vi "Main.vi"() -> ()   [LabVIEW 2018]
doc: "This Continuous Measurement sample project is based on the Queued Message Handler template.\n\nThe Event Handling Loop generates messages based on user interface actions.\n\nThe Message Handling Loop processes messages generated by the Event Handling Loop, or by other messages. There are also Acquisition and Logging message handling loop subVIs, and a chart updating loop."
uses:
  Settings/Settings.ctl
  Acquisition/Hardware Configuration.ctl
  Logging/Logging Configuration.ctl
  controls/UI Data.ctl
  controls/UI State.ctl
  support/Message Queue/Enqueue Message (Single).vi
  <vilib>/Utility/error.llb/Error Cluster From Error Code.vi
  <vilib>/ErrorRing/Error Ring.xnode
  Acquisition/Acquisition.lvlib
  Logging/Logging.lvlib
  Settings/Settings.lvlib
  support/User Event - Stop/User Event - Stop.lvlib
  support/Message Queue/Message Queue.lvlib
panel:
  out "Data":waveform(dbl)[](graph)
  in  "Force Trigger":bool
  in  "Settings":bool
  in  "Start":bool
  in  "Stop":bool
  out "Status":string
  in  "Exit":bool
  # "Continuous Measurement and Logging (NI-DAQmx)"
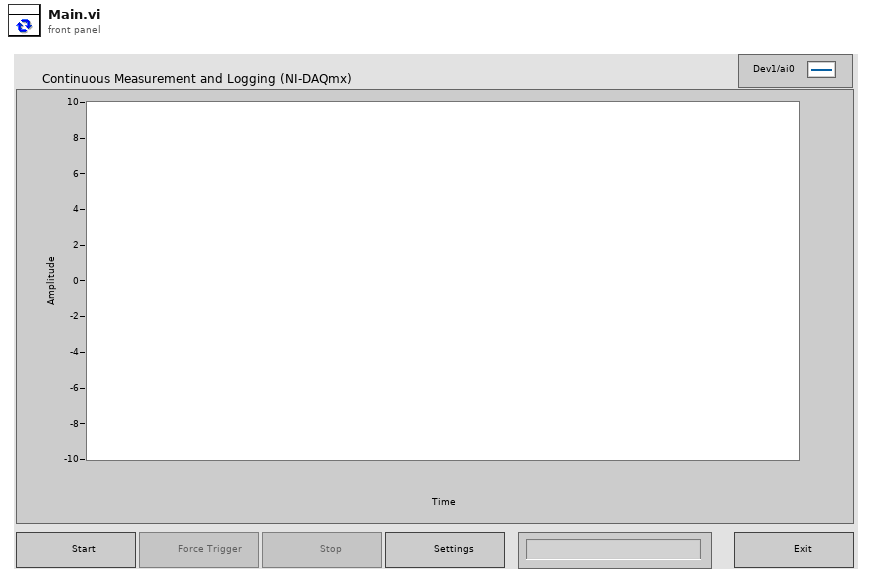
[diagram p1: front panel]
types:
  T1 = typedef "UI State.ctl" = enum16{"Idle", "Acquiring and Logging", "Waiting for Exit", "Waiting for Exit (Acq Stopped)", "Waiting for Exit (Log Stopped)", "Waiting for Stop", "Waiting for Stop (Acq Stopped)", "Waiting for Stop (Log Stopped)"}
  T2 = typedef "UI Data.ctl" = cluster{"Start Ref":refnum<vi>, "Trigger Ref":refnum<vi>, "Stop Ref":refnum<vi>, "Settings Ref":refnum<vi>, "Status Ref":refnum<vi>, "Exit Ref":refnum<vi>, "Data Ref":refnum<vi>}
  T3 = typedef "Settings.lvlib/Settings.ctl" = cluster{"Hardware Configuration":T4, "Logging Configuration":T5}
  T4 = typedef "Acquisition.lvlib/Hardware Configuration.ctl" = cluster{"DAQmx Channel":tag, "Max Input":dbl, "Min Input":dbl, "Sample Rate":dbl, "DAQmx Task":refnum<k21>}
  T5 = typedef "Logging.lvlib/Logging Configuration.ctl" = cluster{"Log File Base Path":path, "TDMS File Reference":refnum<k34>, "Samples to Save":u32, "Trigger - Time":u32, "Trigger - Threshold":dbl, "Trigger - Channel":u32, "Enable Time Trigger":bool, "Enable Threshold Trigger":bool, "Always Log":bool}
  T6 = typedef "Message Queue.lvlib/All Message Queues.ctl" = cluster{"UI":refnum<queue>, "Acquisition":refnum<queue>, "Logging":refnum<queue>}
  T7 = enum8{"Enabled", "Disabled", "Disabled and Grayed Out"}
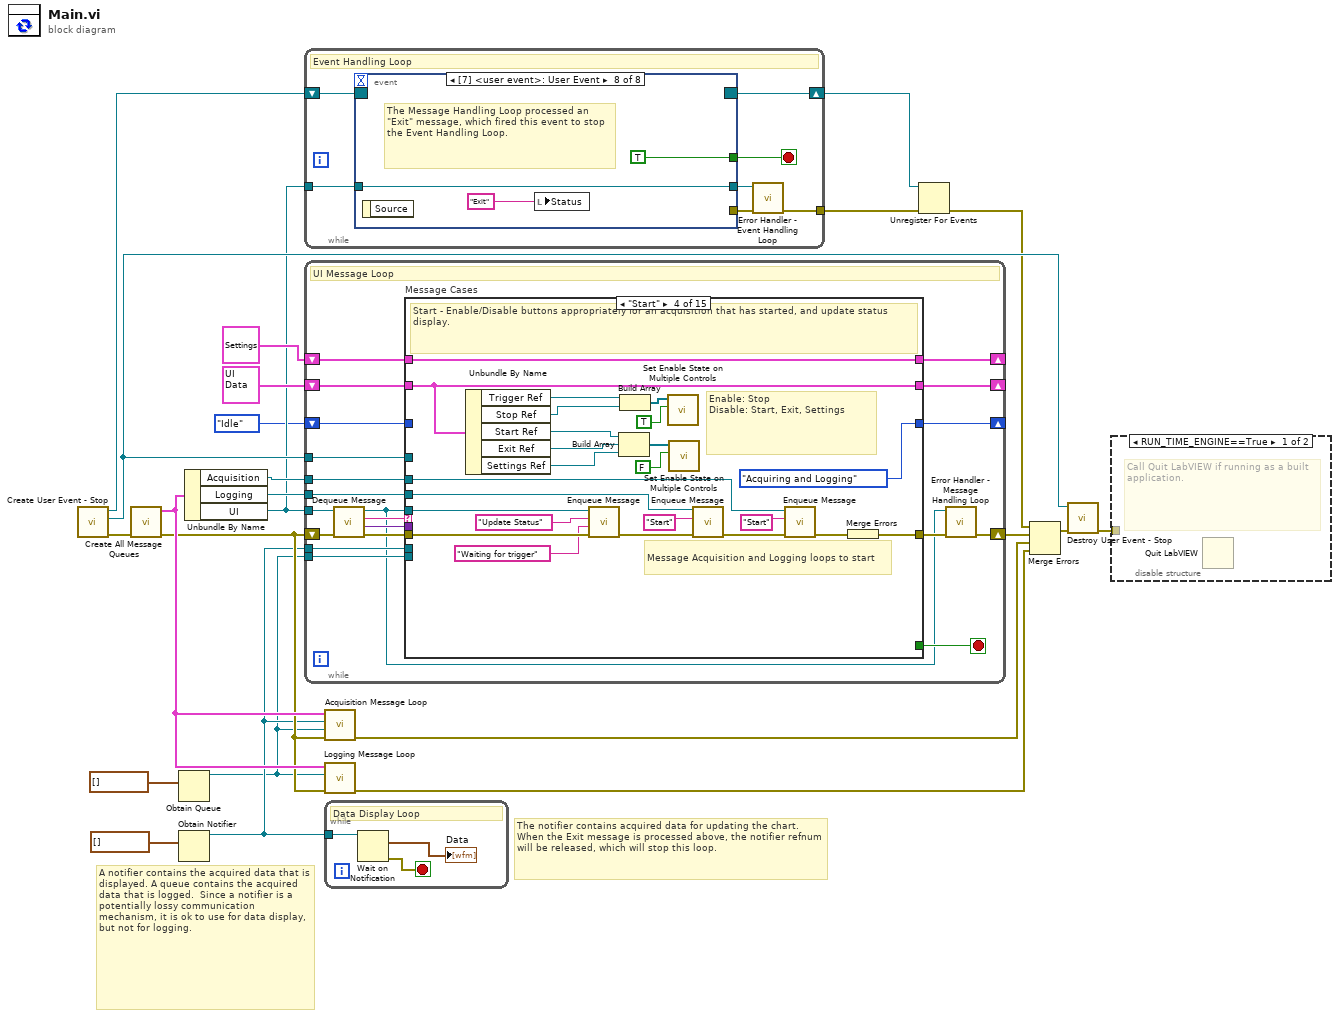
[diagram p0: block diagram]
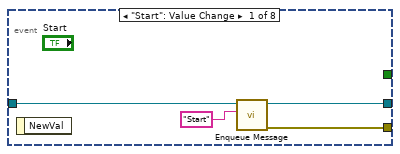
[diagram p3: hidden frame]
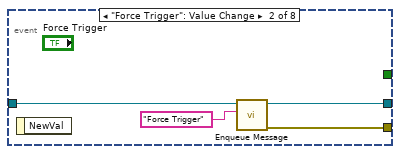
[diagram p4: hidden frame]
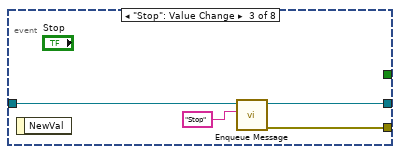
[diagram p5: hidden frame]
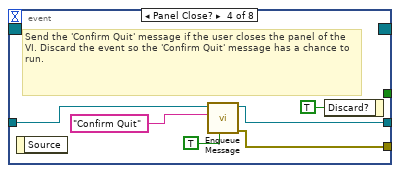
[diagram p6: hidden frame]
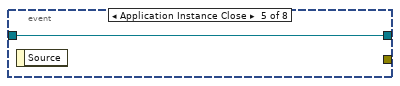
[diagram p7: hidden frame]
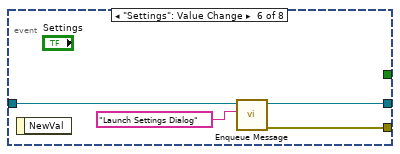
[diagram p8: hidden frame]
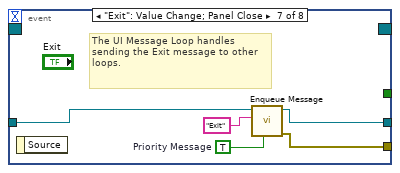
[diagram p9: hidden frame]
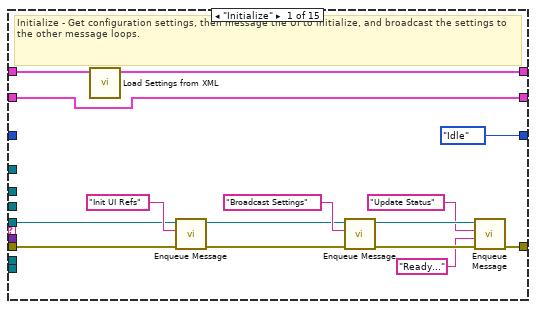
[diagram p10: hidden frame]
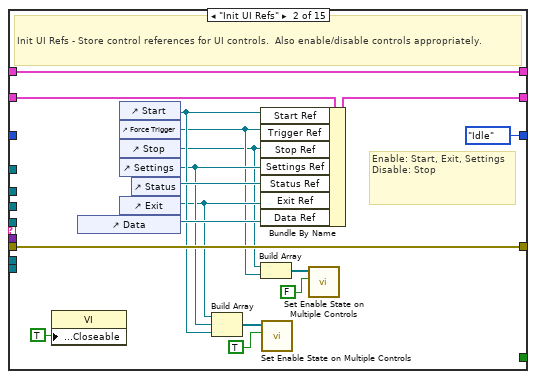
[diagram p11: hidden frame]
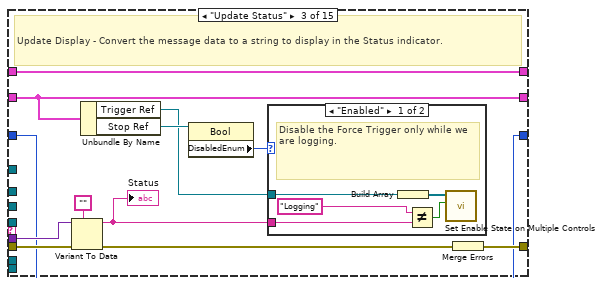
[diagram p12: hidden frame]
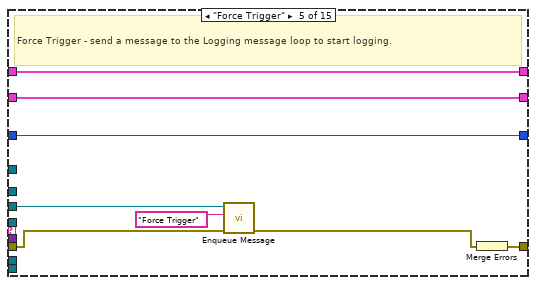
[diagram p14: hidden frame]
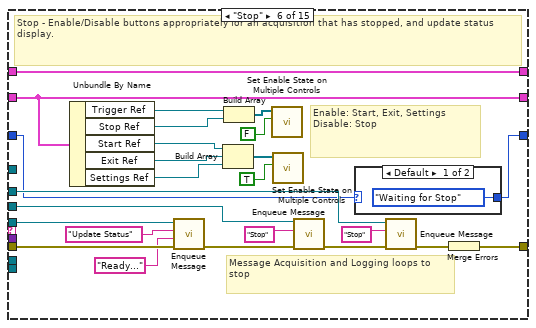
[diagram p15: hidden frame]
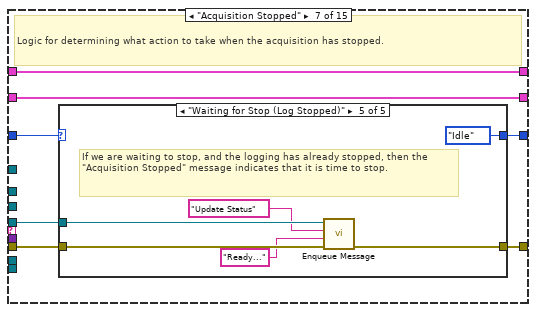
[diagram p17: hidden frame]
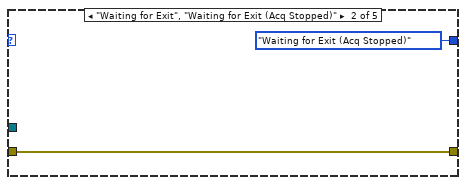
[diagram p19: hidden frame]
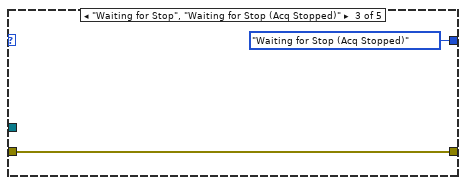
[diagram p20: hidden frame]
diagram:
  # "A notifier contains the acquired data that is displayed. A queue contains the acquired data that is logged.  Since a notifier is a potentially lossy communication mechanism, it is ok to use for data display, but not for logging."
  # "The notifier contains acquired data for updating the chart. When the Exit message is processed above, the notifier refnum will be released, which will stop this loop."
  n1 = call "Create User Event - Stop.vi"() -> ("error out"=w17:errorcluster, "User Event - Stop"=w19:refnum<user-event>, "Stop Event Registration Refnum"=w20:refnum<event-registration>)  [unwired: 9 in]
  n2 = call "Create All Message Queues.vi"("error in (no error)"=w17) -> ("error out"=w14:errorcluster, "Message Queues out"=w16:T6)  [unwired: 9 in]
  n3 = Obtain Queue(element data type=waveform(dbl)[] []) -> (queue out=w3:refnum<queue>)  [unwired: 4 in, 2 out]
  n4 = Obtain Notifier(notification data type=waveform(dbl)[] []) -> (notifier out=w5:refnum<notifier>)  [unwired: 3 in, 2 out]
  n5 = Unbundle By Name(w16) -> ("Acquisition"=w9:refnum<queue>, "Logging"=w8:refnum<queue>, "UI"=w7:refnum<queue>)
  n6 = while {
    tunnel: w7 -> [w29]
    tunnel: [w24] -> w22
    shift-right: [w28] -> w11
    shift-left: w20 -> [w30]
    stop <- w27 stop-if-true
    # "Event Handling Loop"
    n7 = event shown="[7] <user event>: User Event" {
      selector: w30 -> [_ _ _ _ _ _ _ _]
      dyn-events: [_ _ _ _ _ _ _ _] -> w28
      timeout: _ -> [_ _ _ _ _ _ _ _]
      tunnel: [_ _ _ _ _ _ _ TRUE ("Discard?")] -> w27
      tunnel: w29 -> [w32 w37 w41 w48 w49 w51 w55 w59]
      tunnel: [w34 w36 w40 w43 _ w53 w58 _] -> w25
      tunnel: [w31 w35 w39 w44 w49 w50 w54 w59] -> w26
      event "Start": Value Change {
        n8 = event-data() -> ()  [unwired: 1 in, 1 out]
        n9 = call-poly "Enqueue Message.vi"("Message"="Start", "Message Queue"=w32) -> ("error out"=w34:errorcluster, "dup Message Queue"=w31:refnum<queue>)  [unwired: 8 in]
      }
      event "Force Trigger": Value Change {
        n10 = event-data() -> ()  [unwired: 1 in, 1 out]
        n11 = call-poly "Enqueue Message.vi"("Message"="Force Trigger", "Message Queue"=w37) -> ("error out"=w36:errorcluster, "dup Message Queue"=w35:refnum<queue>)  [unwired: 8 in]
      }
      event "Stop": Value Change {
        n12 = event-data() -> ()  [unwired: 1 in, 1 out]
        n13 = call-poly "Enqueue Message.vi"("Message"="Stop", "Message Queue"=w41) -> ("error out"=w40:errorcluster, "dup Message Queue"=w39:refnum<queue>)  [unwired: 8 in]
      }
      event Panel Close? {
        # "Send the 'Confirm Quit' message if the user closes the panel of the VI. Discard the event so the 'Confirm Quit' message has a chance to run."
        n14 = event-data() -> ()  [unwired: 1 in, 1 out]
        n15 = call-poly "Enqueue Message.vi"("Priority Message? (F)"=TRUE, "Message"="Confirm Quit", "Message Queue"=w48) -> ("error out"=w43:errorcluster, "dup Message Queue"=w44:refnum<queue>)  [unwired: 7 in]
        n16 = event-data("Discard?"=TRUE) -> ()  [unwired: 1 in, 1 out]
      }
      event Application Instance Close {
        n17 = event-data() -> ()  [unwired: 1 in, 1 out]
      }
      event "Settings": Value Change {
        n18 = event-data() -> ()  [unwired: 1 in, 1 out]
        n19 = call-poly "Enqueue Message.vi"("Message"="Launch Settings Dialog", "Message Queue"=w51) -> ("error out"=w53:errorcluster, "dup Message Queue"=w50:refnum<queue>)  [unwired: 8 in]
      }
      event "Exit": Value Change; Panel Close {
        w56 = TRUE  # Priority Message
        # "The UI Message Loop handles sending the Exit message to other loops."
        n20 = event-data() -> ()  [unwired: 1 in, 1 out]
        n21 = call-poly "Enqueue Message.vi"("Priority Message? (F)"=w56, "Message"="Exit", "Message Queue"=w55) -> ("error out"=w58:errorcluster, "dup Message Queue"=w54:refnum<queue>)  [unwired: 7 in]
      }
      event User Event {
        # "The Message Handling Loop processed an \"Exit\" message, which fired this event to stop the Event Handling Loop."
        n22 = event-data() -> ()  [unwired: 1 in, 1 out]
        n23 = local write "Status"("Exit" ("Exit String")) -> ()
      }
    }
    n24 = call "Error Handler - Event Handling Loop.vi"("error in (no error)"=w25, "Message Queue"=w26) -> ("dup error in"=w24:errorcluster)  [unwired: 8 in, 1 out]
  }
  n25 = while {
    tunnel: w7 -> [w75]
    tunnel: w19 -> [w80]
    shift-right: [w65] -> w23
    shift-left: w14 -> [w79]
    shift-right: [w74] -> _
    shift-left: T3 {"Hardware Configuration"={"DAQmx Channel"="", "Max Input"=0.0, "Min Input"=0.0, "Sample Rate"=0.0, "DAQmx Task"=""}, "Logging Configuration"={"Log File Base Path"=path "", "TDMS File Reference"=refnum, "Samples to Save"=0, "Trigger - Time"=0, "Trigger - Threshold"=0.0, "Trigger - Channel"=0, "Enable Time Trigger"=FALSE, "Enable Threshold Trigger"=FALSE, "Always Log"=FALSE}} ("Settings") -> [w73]
    shift-right: [w71] -> _
    shift-left: T2 {"Start Ref"=refnum, "Trigger Ref"=refnum, "Stop Ref"=refnum, "Settings Ref"=refnum, "Status Ref"=refnum, "Exit Ref"=refnum, "Data Ref"=refnum} ("Measurement UI Controls") -> [w72]
    tunnel: w9 -> [w70]
    tunnel: w8 -> [w69]
    tunnel: w5 -> [w68]
    tunnel: w3 -> [w67]
    shift-right: [w62] -> _
    shift-left: UI_State."Idle" ("UI State") -> [w63]
    stop <- w81 stop-if-true
    # "UI Message Loop"
    n26 = call "Dequeue Message.vi"("error in (no error)"=w79, "Message Queue"=w75) -> ("error out"=w78:errorcluster, "Message Data"=w76:variant, "Message"=w77:string, "dup Message Queue"=w64:refnum<queue>)  [unwired: 6 in]
    n27 = case "Message Cases" shown="\"Start\"" w77 {
      selector: w77 -> [_ _ _ _ _ _ _ _ _ _ _ _ _ _ w332]
      tunnel: w64 -> [w86 _ _ w153 _ w186 w190 w215 _ w257 w272 w282 w315 _ _]
      tunnel: w78 -> [w85 w113 w124 w152 w159 w185 w192 w217 w245 w259 w276 w281 w323 w330 _]
      tunnel: [w92 w113 w125 w154 w162 w187 w191 w216 w251 w254 w267 w280 w324 w329 w333] -> w66
      tunnel: [_ _ _ _ _ _ _ _ _ _ _ _ TRUE _ _] -> w81
      tunnel: w76 -> [_ _ w123 _ _ _ _ _ _ _ w275 _ _ _ _]
      tunnel: w80 -> [_ _ _ _ _ _ _ _ _ _ _ _ w322 _ _]
      tunnel: [w95 w112 w120 w151 w161 w184 w196 w221 w249 w256 w278 w285 w320 w328 w335] -> w74
      tunnel: w73 -> [w96 w112 w120 w151 w161 w184 w196 w221 w249 w260 w278 w285 w320 w328 w335]
      tunnel: w72 -> [w88 w111 w119 w148 w160 w181 w195 w220 w243 w253 w277 w284 w318 w327 w334]
      tunnel: [w88 w110 w119 w148 w160 w181 w195 w220 w243 w253 w277 w284 w318 w327 w334] -> w71
      tunnel: w70 -> [_ _ _ w135 _ w168 _ _ w242 _ _ _ w317 _ _]
      tunnel: w69 -> [_ _ _ w138 w156 w171 _ _ w241 _ _ _ w316 _ _]
      tunnel: w68 -> [_ _ _ _ _ _ _ _ _ _ _ _ w314 _ _]
      tunnel: w67 -> [_ _ _ _ _ _ _ _ _ _ _ _ w310 _ _]
      tunnel: w63 -> [_ _ w114 _ w155 w164 w194 w219 w240 w252 w266 w283 _ w326 w331]
      tunnel: [UI_State."Idle" ("UI State") UI_State."Idle" ("UI State") w114 UI_State."Acquiring and Logging" ("UI State") w155 w163 w193 w218 w240 w252 w266 w279 UI_State."Idle" ("UI State") w326 w331] -> w62
      frame "Initialize" {
        # "Initialize - Get configuration settings, then message the UI to initialize, and broadcast the settings to the other message loops."
        n28 = call "Load Settings from XML.vi"("Settings in"=w96) -> ("Settings out"=w95:T3)  [unwired: 9 in, 1 out]
        n29 = call-poly "Enqueue Message.vi"("error in (no error)"=w85, "Message"="Init UI Refs", "Message Queue"=w86) -> ("error out"=w83:errorcluster, "dup Message Queue"=w84:refnum<queue>)  [unwired: 7 in]
        n30 = call-poly "Enqueue Message.vi"("error in (no error)"=w83, "Message"="Broadcast Settings", "Message Queue"=w84) -> ("error out"=w94:errorcluster, "dup Message Queue"=w93:refnum<queue>)  [unwired: 7 in]
        n31 = call-poly "Enqueue Message.vi"("error in (no error)"=w94, "Message Data"="Ready..." ("Ready..."), "Message"="Update Status", "Message Queue"=w93) -> ("error out"=w92:errorcluster)  [unwired: 6 in, 1 out]
      }
      frame "Init UI Refs" {
        # "Enable: Start, Exit, Settings\nDisable: Stop"
        # "Init UI Refs - Store control references for UI controls.  Also enable/disable controls appropriately."
        n32 = property class="VI"("Front Panel.Closeable"=TRUE ("Front Panel Window:Closeable")) -> ()  [unwired: 2 in, 2 out]
        n33 = control-ref of="Data"() -> (w106:refnum<vi>)
        n34 = control-ref of="Start"() -> (w105:refnum<vi>)
        n35 = control-ref of="Force Trigger"() -> (w100:refnum<vi>)
        n36 = control-ref of="Stop"() -> (w99:refnum<vi>)
        n37 = control-ref of="Settings"() -> (w102:refnum<vi>)
        n38 = control-ref of="Exit"() -> (w101:refnum<vi>)
        n39 = control-ref of="Status"() -> (w107:refnum<vi>)
        n40 = Build Array(w101, w102, w105) -> (w104:refnum<vi>[])
        n41 = Bundle By Name(cluster=w111, "Start Ref"=w105, "Trigger Ref"=w100, "Stop Ref"=w99, "Settings Ref"=w102, "Status Ref"=w107, "Exit Ref"=w101, "Data Ref"=w106) -> (w110:T2)
        n42 = Build Array(w99, w100) -> (w98:refnum<vi>[])
        n43 = call "Set Enable State on Multiple Controls.vi"("Enable?"=TRUE, "Controls"=w104) -> ()  [unwired: 10 in]
        n44 = call "Set Enable State on Multiple Controls.vi"("Enable?"=FALSE, "Controls"=w98) -> ()  [unwired: 10 in]
      }
      frame "Update Status" {
        # "Update Display - Convert the message data to a string to display in the Status indicator."
        n45 = Variant To Data(error in=w124, type="", Variant=w123) -> (data=w116:string, error out=w121:errorcluster)
        "Status" <- w116
        n46 = Unbundle By Name(w119) -> ("Trigger Ref"=w115:refnum<vi>, "Stop Ref"=w118:refnum<vi>)
        n47 = property class="Bool"(reference=w118) -> ("DisabledEnum"=w117:T7)  [unwired: 1 in, 2 out]
        n48 = case shown="\"Enabled\"" w117 {
          tunnel: w116 -> [w128 _]
          tunnel: w115 -> [w129 _]
          frame "Enabled" {
            # "Disable the Force Trigger only while we are logging."
            n49 = Build Array(w129) -> (w130:refnum<vi>[])
            n50 = Not Equal?(x="Logging" ("Logging"), y=w128) -> (x != y?=w126:bool)
            n51 = call "Set Enable State on Multiple Controls.vi"("Enable?"=w126, "Controls"=w130) -> ()  [unwired: 10 in]
          }
          frame "Disabled", Default {
          }
        }
        n52 = Merge Errors(w121) -> (w125:errorcluster)
      }
      frame "Start" {
        # "Message Acquisition and Logging loops to start"
        # "Enable: Stop\nDisable: Start, Exit, Settings"
        # "Start - Enable/Disable buttons appropriately for an acquisition that has started, and update status display."
        n53 = Unbundle By Name(w148) -> ("Trigger Ref"=w132:refnum<vi>, "Stop Ref"=w133:refnum<vi>, "Start Ref"=w143:refnum<vi>, "Exit Ref"=w142:refnum<vi>, "Settings Ref"=w141:refnum<vi>)
        n54 = call-poly "Enqueue Message.vi"("error in (no error)"=w152, "Message Data"="Waiting for trigger" ("Waiting for trigger"), "Message"="Update Status", "Message Queue"=w153) -> ("error out"=w140:errorcluster)  [unwired: 6 in, 1 out]
        n55 = Build Array(w143, w142, w141) -> (w146:refnum<vi>[])
        n56 = Build Array(w132, w133) -> (w145:refnum<vi>[])
        n57 = call "Set Enable State on Multiple Controls.vi"("Enable?"=TRUE, "Controls"=w145) -> ()  [unwired: 10 in]
        n58 = call "Set Enable State on Multiple Controls.vi"("Enable?"=FALSE, "Controls"=w146) -> ()  [unwired: 10 in]
        n59 = call-poly "Enqueue Message.vi"("error in (no error)"=w140, "Message"="Start", "Message Queue"=w138) -> ("error out"=w137:errorcluster)  [unwired: 7 in, 1 out]
        n60 = call-poly "Enqueue Message.vi"("error in (no error)"=w137, "Message"="Start", "Message Queue"=w135) -> ("error out"=w136:errorcluster)  [unwired: 7 in, 1 out]
        n61 = Merge Errors(w136) -> (w154:errorcluster)
      }
      frame "Force Trigger" {
        # "Force Trigger - send a message to the Logging message loop to start logging."
        n62 = call-poly "Enqueue Message.vi"("error in (no error)"=w159, "Message"="Force Trigger", "Message Queue"=w156) -> ("error out"=w158:errorcluster)  [unwired: 7 in, 1 out]
        n63 = Merge Errors(w158) -> (w162:errorcluster)
      }
      frame "Stop" {
        # "Message Acquisition and Logging loops to stop"
        # "Enable: Start, Exit, Settings\nDisable: Stop"
        # "Stop - Enable/Disable buttons appropriately for an acquisition that has stopped, and update status display."
        n64 = Unbundle By Name(w181) -> ("Trigger Ref"=w165:refnum<vi>, "Stop Ref"=w166:refnum<vi>, "Start Ref"=w176:refnum<vi>, "Exit Ref"=w175:refnum<vi>, "Settings Ref"=w174:refnum<vi>)
        n65 = call-poly "Enqueue Message.vi"("error in (no error)"=w185, "Message Data"="Ready..." ("Ready..."), "Message"="Update Status", "Message Queue"=w186) -> ("error out"=w173:errorcluster)  [unwired: 6 in, 1 out]
        n66 = Build Array(w176, w175, w174) -> (w179:refnum<vi>[])
        n67 = Build Array(w165, w166) -> (w178:refnum<vi>[])
        n68 = call "Set Enable State on Multiple Controls.vi"("Enable?"=FALSE, "Controls"=w178) -> ()  [unwired: 10 in]
        n69 = call "Set Enable State on Multiple Controls.vi"("Enable?"=TRUE, "Controls"=w179) -> ()  [unwired: 10 in]
        n70 = call-poly "Enqueue Message.vi"("error in (no error)"=w173, "Message"="Stop", "Message Queue"=w171) -> ("error out"=w170:errorcluster)  [unwired: 7 in, 1 out]
        n71 = case shown="Default" w164 {
          selector: w164 -> [_ w189]
          tunnel: [UI_State."Waiting for Stop" ("UI State") w189] -> w163
          frame Default {
          }
          frame "Waiting for Exit" {
          }
        }
        n72 = call-poly "Enqueue Message.vi"("error in (no error)"=w170, "Message"="Stop", "Message Queue"=w168) -> ("error out"=w169:errorcluster)  [unwired: 7 in, 1 out]
        n73 = Merge Errors(w169) -> (w187:errorcluster)
      }
      frame "Acquisition Stopped" {
        # "Logic for determining what action to take when the acquisition has stopped."
        n74 = case shown="\"Waiting for Stop (Log Stopped)\"" w194 {
          selector: w194 -> [w198 _ _ _ _]
          tunnel: [w198 UI_State."Waiting for Exit (Acq Stopped)" ("UI State") UI_State."Waiting for Stop (Acq Stopped)" ("UI State") UI_State."Idle" ("UI State") UI_State."Idle" ("UI State")] -> w193
          tunnel: w192 -> [w197 w199 w201 w207 w213]
          tunnel: [w197 w199 w201 w206 w212] -> w191
          tunnel: w190 -> [_ _ _ w205 w211]
          frame Default {
          }
          frame "Waiting for Exit", "Waiting for Exit (Acq Stopped)" {
          }
          frame "Waiting for Stop", "Waiting for Stop (Acq Stopped)" {
          }
          frame "Waiting for Exit (Log Stopped)" {
            # "If we are waiting to exit, and the logging has already stopped, then the \"Acquisition Stopped\" message indicates that it is time to exit."
            n75 = call-poly "Enqueue Message.vi"("Priority Message? (F)"=TRUE, "error in (no error)"=w207, "Message"="Exit", "Message Queue"=w205) -> ("error out"=w206:errorcluster)  [unwired: 6 in, 1 out]
          }
          frame "Waiting for Stop (Log Stopped)" {
            # "If we are waiting to stop, and the logging has already stopped, then the \"Acquisition Stopped\" message indicates that it is time to stop."
            n76 = call-poly "Enqueue Message.vi"("error in (no error)"=w213, "Message Data"="Ready..." ("Message"), "Message"="Update Status", "Message Queue"=w211) -> ("error out"=w212:errorcluster)  [unwired: 6 in, 1 out]
          }
        }
      }
      frame "Logging Stopped" {
        # "Logic for determining what action to take when the logging has stopped."
        n77 = case shown="\"Waiting for Stop (Acq Stopped)\"" w219 {
          selector: w219 -> [w223 _ _ _ _]
          tunnel: [w223 UI_State."Waiting for Exit (Log Stopped)" ("UI State") UI_State."Waiting for Stop (Log Stopped)" ("UI State") UI_State."Idle" ("UI State") UI_State."Idle" ("UI State")] -> w218
          tunnel: w217 -> [w222 w224 w226 w232 w238]
          tunnel: [w222 w224 w226 w231 w237] -> w216
          tunnel: w215 -> [_ _ _ w230 w236]
          frame Default {
          }
          frame "Waiting for Exit", "Waiting for Exit (Log Stopped)" {
          }
          frame "Waiting for Stop", "Waiting for Stop (Log Stopped)" {
          }
          frame "Waiting for Exit (Acq Stopped)" {
            # "If we are waiting to exit, and the acquisition has already stopped, then the \"Logging Stopped\" message indicates that it is time to exit."
            n78 = call-poly "Enqueue Message.vi"("Priority Message? (F)"=TRUE, "error in (no error)"=w232, "Message"="Exit", "Message Queue"=w230) -> ("error out"=w231:errorcluster)  [unwired: 6 in, 1 out]
          }
          frame "Waiting for Stop (Acq Stopped)" {
            # "If we are waiting to stop, and the acquisition has already stopped, then the \"Logging Stopped\" message indicates that it is time to stop."
            n79 = call-poly "Enqueue Message.vi"("error in (no error)"=w238, "Message Data"="Ready..." ("Message"), "Message"="Update Status", "Message Queue"=w236) -> ("error out"=w237:errorcluster)  [unwired: 6 in, 1 out]
          }
        }
      }
      frame "Broadcast settings" {
        w244 = "Update Settings" ("Message")
        # "Send the 'Update Settings' message to the Logging and Acquisition message loops."
        n80 = Unbundle By Name(w249) -> ("Hardware Configuration"=w248:T4, "Logging Configuration"=w247:T5)
        n81 = call-poly "Enqueue Message.vi"("Message Data"=w248, "Message"=w244, "Message Queue"=w242) -> ("error out"=w250:errorcluster)  [unwired: 7 in, 1 out]
        n82 = call-poly "Enqueue Message.vi"("error in (no error)"=w250, "Message Data"=w247, "Message"=w244, "Message Queue"=w241) -> ("error out"=w246:errorcluster)  [unwired: 6 in, 1 out]
        n83 = Merge Errors(w246, w245) -> (w251:errorcluster)
      }
      frame "Launch Settings Dialog" {
        # "Launch the Settings Dialog when the user clicks the 'Settings' button."
        n84 = call "Settings Dialog.vi"("error in (no error)"=w259, "Settings in"=w260) -> ("error out"=w255:errorcluster, "Cancelled?"=w258:bool, "Settings out"=w256:T3)  [unwired: 6 in, 1 out]
        n85 = case shown="False" w258 {
          tunnel: w257 -> [w264 _]
          tunnel: w255 -> [w263 w265]
          tunnel: [w262 w265] -> w254
          frame False {
            n86 = call-poly "Enqueue Message.vi"("error in (no error)"=w263, "Message"="Broadcast Settings", "Message Queue"=w264) -> ("error out"=w262:errorcluster)  [unwired: 7 in, 1 out]
          }
          frame True {
          }
        }
      }
      frame "Error" {
        # "Error - Check the error message data and respond accordingly. This message is sent by the \"Error Handler\" VIs at the end of each loop in this application."
        n87 = Variant To Data(error in=w276, type=errorcluster {"status"=FALSE, "code"=0, "source"=""} ("error out"), Variant=w275) -> (data=w273:errorcluster, error out=w269:errorcluster)
        n88 = call <vilib>:"Simple Error Handler.vi"("error in (no error)"=w273) -> ()  [unwired: 4 in, 5 out]
        n89 = call-poly "Enqueue Message.vi"("Priority Message? (F)"=TRUE, "Message"="Exit", "Message Queue"=w272) -> ("error out"=w268:errorcluster)  [unwired: 7 in, 1 out]
        n90 = Merge Errors(w268, w269) -> (w267:errorcluster)
      }
      frame "Confirm Quit" {
        # "Confirm Quit - Message that can confirm whether or not the user wants to exit the application."
        n91 = case shown="\"Acquiring and Logging\"" w283 {
          tunnel: w282 -> [w290 w296]
          tunnel: w281 -> [w289 w294]
          tunnel: [w286 w293] -> w280
          tunnel: [UI_State."Idle" ("UI State") w292] -> w279
          frame Default {
            # "If 'Confirm Quit' comes in while the system is idle, there is no need for a confirmation message."
            n92 = call-poly "Enqueue Message.vi"("Priority Message? (F)"=TRUE, "error in (no error)"=w289, "Message"="Exit", "Message Queue"=w290) -> ("error out"=w286:errorcluster)  [unwired: 6 in, 1 out]
          }
          frame "Acquiring and Logging" {
            n93 = Two Button Dialog(message="Are you sure you want to quit while the acquisition is running?" ("Confirm Quit Message"), 1:"No" ("No"), 2:"Yes" ("Yes")) -> (T button?=w295:bool)
            n94 = case shown="True" w295 {
              tunnel: w296 -> [_ w306]
              tunnel: w294 -> [w300 w305]
              tunnel: [w300 w304] -> w293
              tunnel: [UI_State."Acquiring and Logging" ("UI State") UI_State."Waiting for Exit" ("UI State")] -> w292
              frame False {
                # "User did not want to quit."
              }
              frame True {
                n95 = call-poly "Enqueue Message.vi"("error in (no error)"=w305, "Message"="Stop", "Message Queue"=w306) -> ("error out"=w304:errorcluster)  [unwired: 7 in, 1 out]
              }
            }
          }
        }
      }
      frame "Exit" {
        w319 = "Exit" ("Message")
        # "Don't check the error outs. The acquisition and logging queues may have already been released."
        # "Close references owned by the Main VI."
        # "Stop the VI"
        # "Exit - Fire the User Event to stop the Event Handling Loop.  Also send Exit messages to the Acquisition and Logging loops."
        n96 = Release Queue(queue=w315, error in (no error)=w323) -> (error out=w313:errorcluster)  [unwired: 1 in, 2 out]
        n97 = call "Fire User Event - Stop.vi"("User Event - Stop"=w322) -> ("error out"=w321:errorcluster)  [unwired: 10 in]
        n98 = Release Notifier(notifier=w314, error in (no error)=w313) -> (error out=w312:errorcluster)  [unwired: 1 in, 2 out]
        n99 = Release Queue(queue=w310, error in (no error)=w312) -> (error out=w311:errorcluster)  [unwired: 1 in, 2 out]
        n100 = call-poly "Enqueue Message.vi"("Priority Message? (F)"=TRUE, "Message"=w319, "Message Queue"=w317) -> ()  [unwired: 7 in, 2 out]
        n101 = call-poly "Enqueue Message.vi"("Priority Message? (F)"=TRUE, "Message"=w319, "Message Queue"=w316) -> ()  [unwired: 7 in, 2 out]
        n102 = Merge Errors(w321, w311) -> (w324:errorcluster)
      }
      frame "---Copy This Frame---" {
        # "Duplicate this frame when creating new messages.  Change this comment in the duplicated frame to describe this message."
        n103 = Merge Errors(w330) -> (w329:errorcluster)
      }
      frame Default {
        # "'Default' case only runs if there is a message that isn't defined in any of the other cases.  Output a programming error."
        n104 = xnode "Error Ring"("parameter 0"=w332) -> ("error out"=w333:errorcluster)
      }
    }
    n105 = call "Error Handler - Message Handling Loop.vi"("error in (no error)"=w66, "Message Queue"=w64) -> ("dup error in"=w65:errorcluster)  [unwired: 8 in, 1 out]
  }
  n106 = call "Acquisition Message Loop.vi"("error in (no error)"=w14, "Data Queue"=w3, "Data Notifier"=w5, "Message Queues"=w16) -> ("error out"=w18:errorcluster)  [unwired: 7 in]
  n107 = call "Logging Message Loop.vi"("error in (no error)"=w14, "Data Queue"=w3, "Message Queues"=w16) -> ("error out"=w15:errorcluster)  [unwired: 8 in]
  n108 = while "Data Display Loop" {
    tunnel: w5 -> [w345]
    stop <- w343 stop-if-true
    # "Data Display Loop"
    n109 = Wait on Notification(notifier=w345) -> (notification=→"Data":waveform(dbl)[], error out=w343:errorcluster)  [unwired: 3 in, 2 out]
  }
  n110 = Unregister For Events(event registration refnum=w11, error in=w22) -> (error out=w12:errorcluster)
  n111 = Merge Errors(w12, w23, w18, w15) -> (w21:errorcluster)
  n112 = call "Destroy User Event - Stop.vi"("error in (no error)"=w21, "User Event - Stop"=w19) -> ("error out"=w2:errorcluster)  [unwired: 9 in]
  n113 = disable-structure shown="RUN_TIME_ENGINE==True" {
    disable-tunnel: w2 -> [_ _]
    frame condition #0 {
      # "Call Quit LabVIEW if running as a built application."
      n114 = Quit LabVIEW() -> ()  [unwired: 1 in]
    }
    frame condition #1 (active) {
    }
  }
